vi "RESET SparkMAX motor.vi"(8 "error in (no error)":errorcluster, 11 "SparkMAX motor refname":string="My Motor RefNum") -> (0 "error out":errorcluster, 1 "RESET success?":bool, 2 "Sensor Position":dbl, 3 "MotorControlDevRef out":T1)   [LabVIEW 2020]
uses:
  <vilib>/Rock Robotics/WPI/MotorControl/WPI_MotorControlDeviceRef.ctl
  <vilib>/Rock Robotics/WPI/MotorControl/WPI_MotorControlType.ctl
  <vilib>/Rock Robotics/SystemInterfaces/DIO/FPGA_DIOPWMChannel.ctl
  <vilib>/Rock Robotics/WPI/PWM/WPI_PWMDeadband.ctl
  <vilib>/Rock Robotics/SystemInterfaces/DIO/FPGA_DIOChannel.ctl
  <vilib>/Rock Robotics/WPI/ThirdParty/REV Robotics/REVLib/Typedef/Spark MAX Sensor Type.ctl
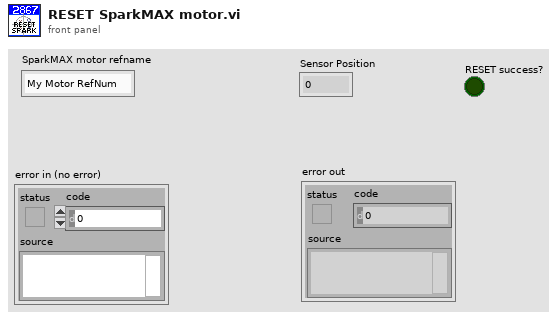
[diagram p1: front panel]
types:
  T1 = typedef "WPI_MotorControlDeviceRef.ctl" = cluster{"DeviceStatus":errorcluster, "Type":T2, "PWM":cluster{"PWM Channel":T3, "DeadBand":T4}, "CAN":cluster{"Device Number":u8, "SetOutput VI Ref":variant, "GetOutput VI Ref":variant, "Enable VI Ref":variant, "Disable VI Ref":variant, "Data":variant}, "Invert":bool, "DIO PWM":cluster{"PWM \"Enable\" Channel":T3, "DIOChannel":T5, "PWM Rate":dbl}}
  T2 = typedef "WPI_MotorControlType.ctl" = enum16{"PWM", "CAN", "DIO PWM"}
  T3 = typedef "FPGA_DIOPWMChannel.ctl" = enum8{"PWM 0", "PWM 1", "PWM 2", "PWM 3", "PWM 4", "PWM 5", "PWM 6", "PWM 7", "PWM 8", "PWM 9", "PWM MXP 0", "PWM MXP 1", "PWM MXP 2", "PWM MXP 3", "PWM MXP 4", "PWM MXP 5", "PWM MXP 6", "PWM MXP 7", "PWM MXP 8", "PWM MXP 9", "Invalid"}
  T4 = typedef "WPI_PWMDeadband.ctl" = cluster{"Name":string, "maxPositivePwm":i32, "minPositivePwm":i32, "centerPwm":i32, "maxNegativePwm":i32, "minNegativePwm":i32, "angularRange":u16}
  T5 = typedef "FPGA_DIOChannel.ctl" = enum8{"DIO 0", "DIO 1", "DIO 2", "DIO 3", "DIO 4", "DIO 5", "DIO 6", "DIO 7", "DIO 8", "DIO 9", "DIO MXP 0", "DIO MXP 1", "DIO MXP 2", "DIO MXP 3", "DIO MXP 4", "DIO MXP 5", "DIO MXP 6", "DIO MXP 7", "DIO MXP 8", "DIO MXP 9", "DIO MXP 10", "DIO MXP 11", "DIO MXP 12", "DIO MXP 13", "DIO MXP 14", "DIO MXP 15", "SPI Port CS1", "SPI Port CS2", "SPI Port CS3", "SPI Port MISO", "SPI Port MOSI", "Invalid"}
  T6 = typedef "Spark MAX Sensor Type.ctl" = enum16{"No Sensor", "Hall Sensor", "Encoder", "-Not Available-", "Analog", "Alternate Encoder"}
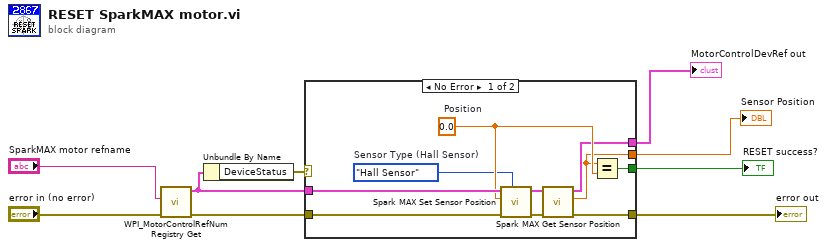
[diagram p0: block diagram]
diagram:
  n1 = call <vilib>:"WPI_MotorControlRefNum Registry Get.vi"("error in (no error)"="error in (no error)", "refnum name"="SparkMAX motor refname") -> ("error out"=w9:errorcluster, "MotorControlDevRef"=w2:T1)  [unwired: 8 in]
  n2 = Unbundle By Name(w2) -> ("DeviceStatus"=w1:errorcluster)
  n3 = case shown="No Error" w1 {
    tunnel: w9 -> [w19 _]
    tunnel: w2 -> [w18 _]
    tunnel: [w15 _] -> w7
    tunnel: [w13 _] -> w6
    tunnel: [w12 _] -> w4
    tunnel: [w11 _] -> w3
    frame No Error {
      w10 = Spark_MAX_Sensor_Type."Hall Sensor"  # Sensor Type (Hall Sensor)
      w14 = 0.0  # Position
      n4 = call <vilib>:"Spark MAX Set Sensor Position.vi"("Sensor Type (Hall Sensor)"=w10, "error in"=w19, "Position"=w14, "MotorControlDeviceRef"=w18) -> ("error out"=w16:errorcluster, "MotorControlDeviceRef"=w17:T1)  [unwired: 6 in]
      n5 = call <vilib>:"Spark MAX Get Sensor Position.vi"("error in (no error)"=w16, "MotorControlDevRef in"=w17) -> ("error out"=w15:errorcluster, "Sensor Position"=w12:dbl, "MotorControlDevRef out"=w11:T1)  [unwired: 6 in, 1 out]
      n6 = Equal?(x=w12, y=w14) -> (x = y?=w13:bool)
    }
    frame Error {
    }
  }
  "Sensor Position" <- w4
  "error out" <- w7
  "RESET success?" <- w6
  "MotorControlDevRef out" <- w3
